vi "PH_Img_BaseClass.set Camera Instancename.vi"(0 "i ref in":refnum<vi>, 2 "Camera Instancename":string, 5 "error in (no error)":errorcluster) -> (14 "i ref out":refnum<vi>, 19 "error out":errorcluster)   [LabVIEW 2014, in "PH_Img_BaseClass.lvlib"]
uses:
  PH_Img_BaseClass.lvlib
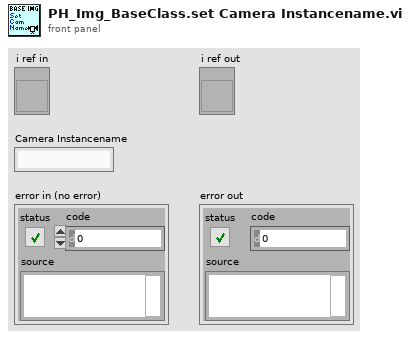
[diagram p1: front panel]
types:
  T1 = typedef "PH_Img_BaseClass.lvlib/PH_Img_BaseClass.i attribute.ctl" = cluster{"GUI Refs":T2, "Timeout Image [ms]":i32, "Default Periodic Period [ms]":i32, "Camera":cluster{"Instancename":string, "Notifier":refnum<notifier>}, "Palette":T3, "Cam Settings":cluster{"Cam ID":string, "Gain":dbl, "Brightness":dbl, "Shutter":dbl, "Cam Info Failure":bool, "Mode":i32}}
  T2 = typedef "PH_Img_BaseClass.lvlib/PH_Img_BaseClass.GUI Refs.ctl" = cluster{"Timeout":refnum<vi>, "Image":refnum<vi>, "Palette":refnum<vi>, "Timeout Set":refnum<vi>}
  T3 = typedef "PH_Img_BaseClass.lvlib/PH_Img_BaseClass.Palette.ctl" = i32
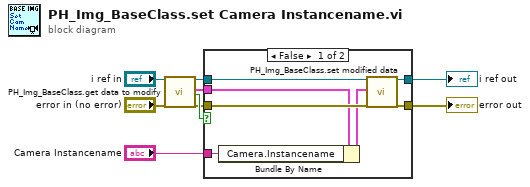
[diagram p0: block diagram]
diagram:
  n1 = call "PH_Img_BaseClass.get data to modify.vi"("i ref in"="i ref in", "error in (no error)"="error in (no error)") -> ("i ref out"=w6:refnum<vi>, "i attribute"=w7:T1, "timed out"=w8:bool, "error out"=w4:errorcluster)  [unwired: 14 in]
  n2 = case shown="False" w8 {
    tunnel: [w16 w18] -> w1
    tunnel: [w15 w17] -> w3
    tunnel: w4 -> [w14 w17]
    tunnel: w6 -> [w13 w18]
    tunnel: w7 -> [w12 _]
    tunnel: "Camera Instancename" -> [w10 _]
    frame False {
      n3 = Bundle By Name(cluster=w12, "Camera.Instancename"=w10) -> (w11:T1)
      n4 = call "PH_Img_BaseClass.set modified data.vi"("i ref in"=w13, "i attribute"=w11, "error in (no error)"=w14) -> ("i ref out"=w16:refnum<vi>, "error out"=w15:errorcluster)  [unwired: 15 in]
    }
    frame True {
    }
  }
  "error out" <- w3
  "i ref out" <- w1
